vi "CreateEvents.vi"() -> (0 "error out":errorcluster, 3 "Events":T1)   [LabVIEW 2015]
uses:
  TypeDef/EventsReference.ctl
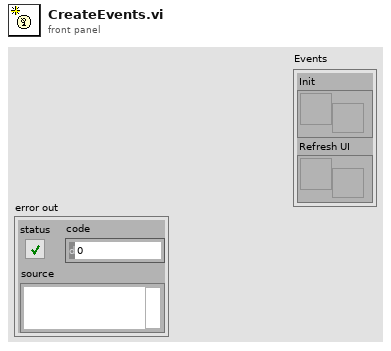
[diagram p1: front panel]
types:
  T1 = typedef "EventsReference.ctl" = cluster{"Init":refnum<user-event>, "Refresh UI":refnum<user-event>}
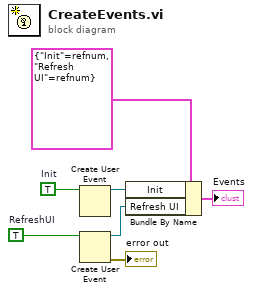
[diagram p0: block diagram]
diagram:
  w7 = TRUE  # Init
  w6 = TRUE  # RefreshUI
  n1 = Create User Event(user event datatype=w7) -> (user event=w2:refnum<user-event>)  [unwired: 1 in, 1 out]
  n2 = Create User Event(user event datatype=w6) -> (user event=w1:refnum<user-event>, error out=→"error out":errorcluster)  [unwired: 1 in]
  n3 = Bundle By Name(cluster=T1 {"Init"=refnum, "Refresh UI"=refnum} ("Cluster"), "Init"=w2, "Refresh UI"=w1) -> (→"Events":T1)
